vi "SortByName.vi"(8 "error in (no error)":errorcluster, 10 "Sort by":string, 11 "Products":T1[](array[typedef])) -> (0 "error out":errorcluster, 3 "Sorted Products":T1[](array[typedef]))   [LabVIEW 2022 SP3]
uses:
  25408b5c-fc92-4fea-9d8a-3ba5747587d2.vi
  #typedef_product.ctl
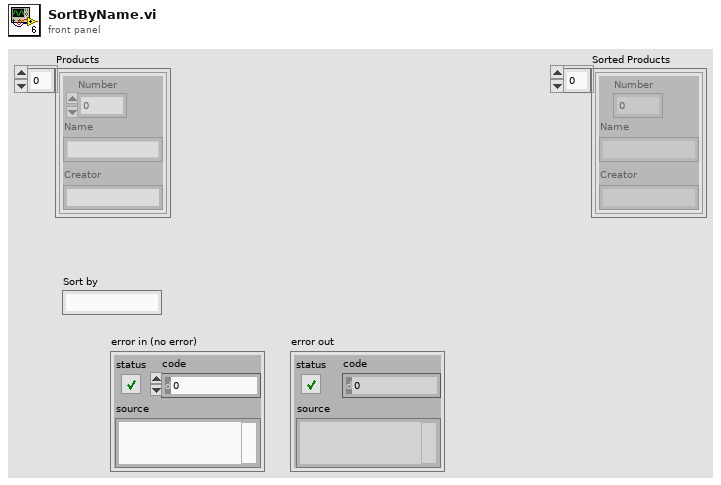
[diagram p1: front panel]
types:
  T1 = typedef "#typedef_product.ctl" = cluster{"Number ":i32, "Name":string, "Creator":string}
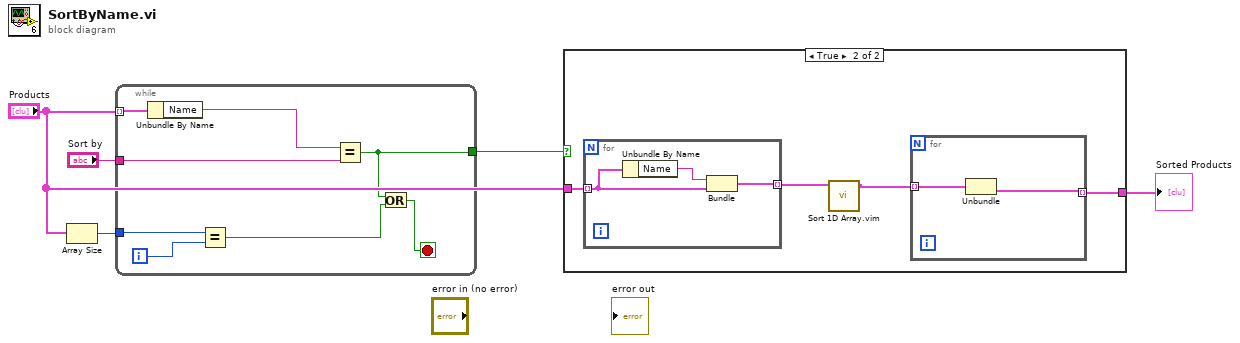
[diagram p0: block diagram]
diagram:
  n1 = Array Size(array="Products") -> (size(s)=w4:i32)
  n2 = while {
    tunnel: "Products" -> [w13] mode=indexing
    tunnel: w4 -> [w12]
    tunnel: [w8] -> w3
    tunnel: "Sort by" -> [w6]
    i -> [w11]
    stop <- w9 stop-if-true
    n3 = Unbundle By Name(w13) -> ("Name"=w7:string)
    n4 = Equal?(x=w12, y=w11) -> (x = y?=w10:bool)
    n5 = Equal?(x=w7, y=w6) -> (x = y?=w8:bool)
    n6 = Or(x=w8, y=w10) -> (x .or. y?=w9:bool)
  }
  n7 = case shown="True" w3 {
    tunnel: [w14 w16] -> w2
    tunnel: "Products" -> [w14 w15]
    frame False {
    }
    frame True {
      n8 = for {
        tunnel: w15 -> [w22] mode=indexing
        tunnel: [w21] -> w18 mode=indexing
        n9 = Unbundle By Name(w22) -> ("Name"=w23:string)
        n10 = Bundle("Name"=w23, "Product"=w22) -> (w21:cluster{"Name":string, "Product":T1})  [unwired: 1 in]
      }
      n11 = call "Sort 1D Array.vim"("unsorted array"=w18) -> ("sorted array"=w17:cluster{"Name":string, "Product":T1}[])  [unwired: 10 in]
      n12 = for {
        tunnel: w17 -> [w20] mode=indexing
        tunnel: [w19] -> w16 mode=indexing
        n13 = Unbundle(w20) -> ("Product"=w19:T1)  [unwired: 1 out]
      }
    }
  }
  "Sorted Products" <- w2
